vi "Read Actuator Settings.vi"(8 "error in (no error)":errorcluster, 11 "Boot Loader in":refnum<class "Boot Loader.lvclass">) -> (0 "error out":errorcluster, 2 "FASettings":T1, 3 "Boot Loader out":refnum<class "Boot Loader.lvclass">)   [LabVIEW 2015, in "Boot Loader.lvclass"]
uses:
  Boot Loader.lvclass
  Common_RT_FAILC/DataTypes/FASettings.ctl
  Common_RT_ILC/DataTypes/ILCSettings.ctl
  Common_RT_FAILC/DataTypes/FATypes.ctl
  Settings/Settings.lvclass
  Common_RT_ILC/RTILC.lvlib
  Common_RT_FAILC/RTFAILC.lvlib
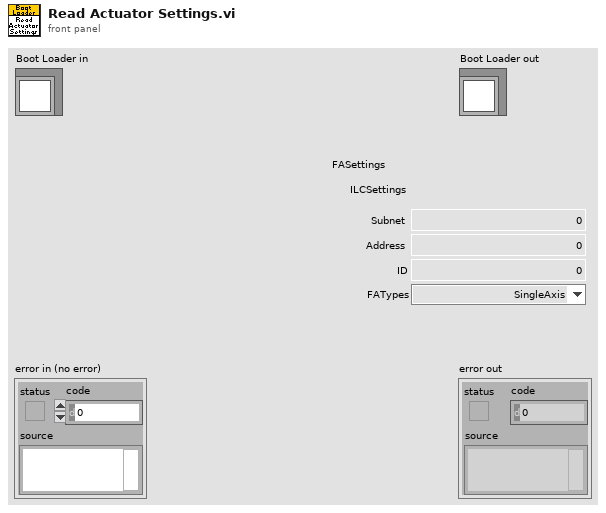
[diagram p1: front panel]
types:
  T1 = typedef "RTFAILC.lvlib/FASettings.ctl" = cluster{"ILCSettings":T2, "ID":i16, "FATypes":T3}
  T2 = typedef "RTILC.lvlib/ILCSettings.ctl" = cluster{"Subnet":u8, "Address":u8}
  T3 = typedef "RTFAILC.lvlib/FATypes.ctl" = enum16{"SingleAxis", "LateralDualAxis", "CrossLateralDualAxis"}
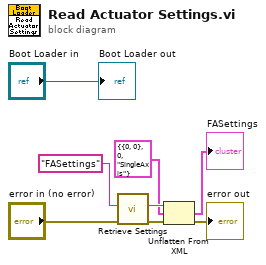
[diagram p0: block diagram]
diagram:
  n1 = call "Retrieve Settings.vi"("error in (no error)"="error in (no error)", "configName"="FASettings") -> ("error out"=w4:errorcluster, "xmlConfig"=w7:string)  [unwired: 7 in, 1 out]
  n2 = Unflatten From XML(xml string=w7, type=T1 {"ILCSettings"={"Subnet"=0, "Address"=0}, "ID"=0, "FATypes"=enum."SingleAxis"} ("FASettings"), error in (no error)=w4) -> (value=→"FASettings":T1, error out=→"error out":errorcluster)
  "Boot Loader out" <- "Boot Loader in"
